vi "DemoServer.vi"() -> ()   [LabVIEW 2019]
panel:
  out "Array":string[](array[string])
  out "IP Address":string
  in  "stop":bool
  out "Position":string
  in  "Joints":T1(array[cluster])=[{"Theta (degrees)"=-23.636363636363654, "d"=1.6, "a"=0.0, "alpha (degrees)"=-90.0}, {"Theta (degrees)"=38.18181818181819, "d"=0.0, "a"=1.0, "alpha (degrees)"=0.0}, {"Theta (degrees)"=-49.09090909090909, "d"=0.0, "a"=1.0, "alpha (degrees)"=0.0}, {"Theta (degrees)"=-27.27272727272728, "d"=0.0, "a"=0.7, "alpha (degrees)"=0.0}] {"alpha (degrees)" format="%.2f"; "a" format="%.2f"; "d" format="%.2f"; "Theta (degrees)" scale=-180.0..180.0}
  out "3D Picture":refnum<vi>(3d-picture)
  out "data":string
  # ":5002"
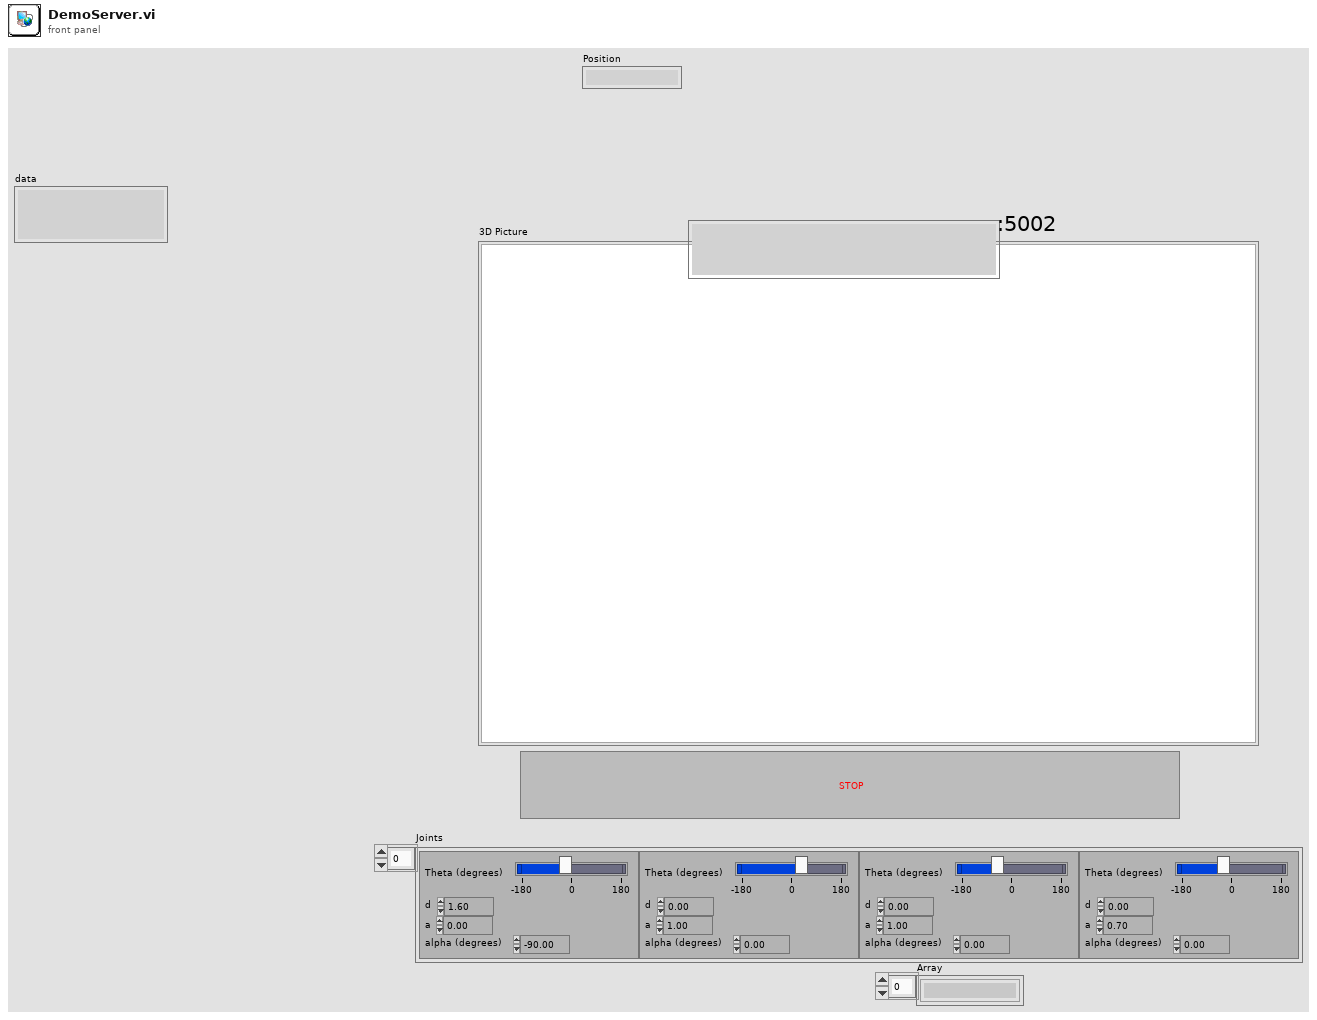
[diagram p1: front panel]
types:
  T1 = cluster{"Theta (degrees)":dbl, "d":dbl, "a":dbl, "alpha (degrees)":dbl}[]
  T2 = enum16{"Standard", "Buffered", "CRLF", "Immediate"}
  T3 = cluster{"Theta (degrees)":dbl, "d":dbl, "a":dbl, "alpha (degrees)":dbl}
  T4 = cluster{"Line width":sgl, "Line Color":u32, "Axes?":bool}
  T5 = typedef "NI_Matrix.lvlib/RealMatrix.ctl" = dbl[][]
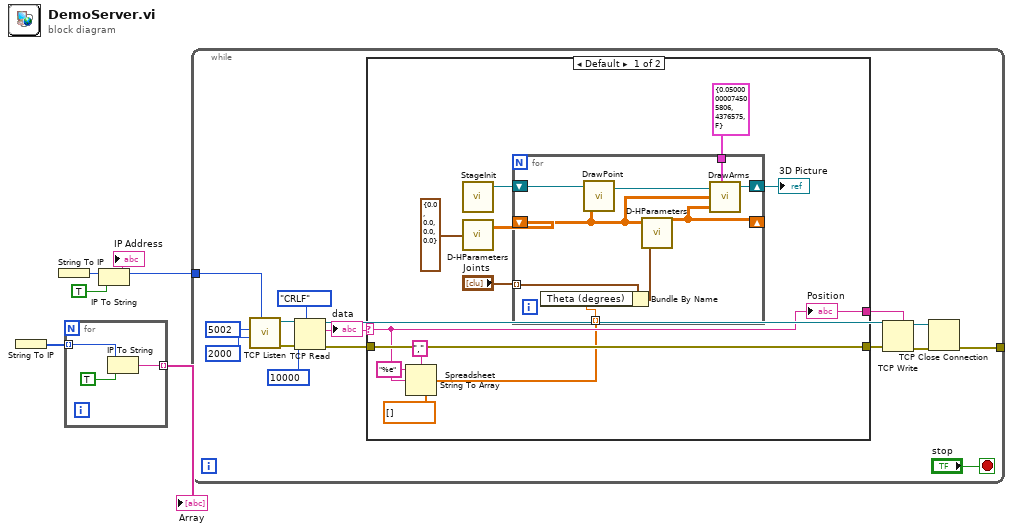
[diagram p0: block diagram]
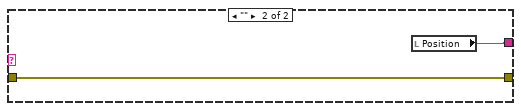
[diagram p2: hidden frame]
diagram:
  n1 = String To IP() -> (0:w3:u32[])  [unwired: 1 in]
  n2 = String To IP() -> (0:w1:u32)  [unwired: 1 in]
  n3 = for {
    tunnel: w3 -> [w7] mode=indexing
    tunnel: [w6] -> w2 mode=indexing
    n4 = IP To String(1:TRUE ("dot notation? (F)"), 2:w7) -> (0:w6:string)
  }
  "Array" <- w2
  n5 = IP To String(1:TRUE ("dot notation? (F)"), 2:w1) -> (0:→"IP Address":string)
  n6 = while {
    tunnel: [w11] -> _
    tunnel: w1 -> [w9]
    stop <- "stop" stop-if-true
    n7 = call <vilib>:"TCP Listen.vi"("net address"=w9, "timeout ms (wait forever: -1)"=2000, "port"=u16 5002) -> ("error out"=w15:errorcluster, "connection ID"=w16:refnum<k5>)  [unwired: 4 in, 3 out]
    n8 = TCP Read(connection ID=w16, bytes to read=10000, error in (no error)=w15, 7:T2."CRLF" ("mode (standard)")) -> (connection ID out=w19:refnum<k5>, data out=w18:string, error out=w20:errorcluster)  [unwired: 1 in]
    "data" <- w18
    n9 = case shown="Default" w18 {
      selector: w18 -> [w29 _]
      tunnel: w20 -> [w36 w47]
      tunnel: [w36 w47] -> w21
      tunnel: [w29 w46] -> w13
      frame Default {
        n10 = Spreadsheet String To Array(delimiter (Tab)=",", format string="%e", spreadsheet string=w29, array type (2D Dbl)=dbl[] []) -> (array=w25:dbl[])
        n11 = call <userlib>:"StageInit.vi"() -> ("Stage out"=w32:refnum<vi>)  [unwired: 4 in, 1 out]
        n12 = call <userlib>:"D-HParameters.vi"("n+1"=T3 {"Theta (degrees)"=0.0, "d"=0.0, "a"=0.0, "alpha (degrees)"=0.0}) -> ("A x B"=w30:T5)  [unwired: 2 in]
        n13 = for {
          shift-right: [w44] -> _
          shift-left: w30 -> [w40]
          tunnel: "Joints" -> [w39] mode=indexing
          tunnel: T4 {"Line width"=0.05, "Line Color"=4376575, "Axes?"=FALSE} ("Params") -> [w45]
          shift-right: [w43] -> w33
          shift-left: w32 -> [w42]
          tunnel: w25 -> [w38] mode=indexing
          n14 = Bundle By Name(cluster=w39, "Theta (degrees)"=w38) -> (w37:T3)
          n15 = call <userlib>:"DrawPoint.vi"("Start"=w40, "Stage in"=w42) -> ("Stage out"=w41:refnum<vi>)  [unwired: 1 in]
          n16 = call <userlib>:"D-HParameters.vi"("n+1"=w37, "Start"=w40) -> ("A x B"=w44:T5)  [unwired: 1 in]
          n17 = call <userlib>:"DrawArms.vi"("Stage in"=w41, "Params"=w45, "Start"=w40, "End"=w44) -> ("Stage out"=w43:refnum<vi>)  [unwired: 2 in, 1 out]
        }
        "3D Picture" <- w33
        "Position" <- w29
      }
      frame "" {
        n18 = local read "Position"() -> (w46:string)
      }
    }
    n19 = TCP Write(connection ID=w19, data in=w13, error in (no error)=w21) -> (connection ID out=w23:refnum<k5>, error out=w22:errorcluster)  [unwired: 1 in, 1 out]
    n20 = TCP Close Connection(connection ID=w23, error in (no error)=w22) -> (error out=w11:errorcluster)  [unwired: 1 in, 1 out]
  }
